vi "ConvertTimes - Array.vi"(1 "GP22 results":dbl[](array[numeric])) -> (0 "Array of times / s":dbl[](array[numeric]))   [LabVIEW 2017, in "GP22_TDC_Arduinoed.lvlib"]
doc: "Convert fixed point output of GP22 to time value in seconds."
uses:
  GP22_TDC_Arduinoed.lvlib
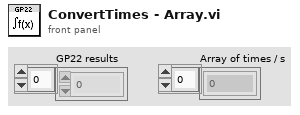
[diagram p1: front panel]
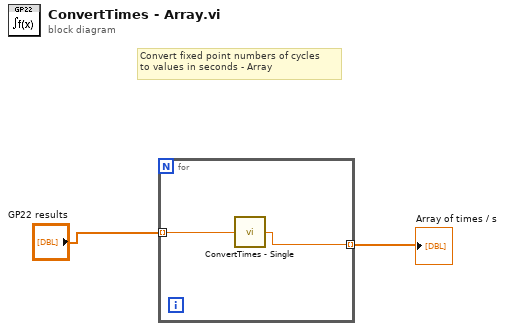
[diagram p0: block diagram]
diagram:
  # "Convert fixed point numbers of cycles\nto values in seconds - Array"
  n1 = for {
    tunnel: "GP22 results" -> [w4] mode=indexing
    tunnel: [w3] -> w1 mode=indexing
    n2 = call "ConvertTimes - Single.vi"("GP22 Output"=w4) -> ("Time/s"=w3:dbl)
  }
  "Array of times / s" <- w1
